vi "HTTP URL Format.vi"(3 "Endpoint":string="/Status", 4 "Port":string="11200", 5 "IP Address":string="10.0.40.4") -> (2 "URL":string)   [LabVIEW 2020]
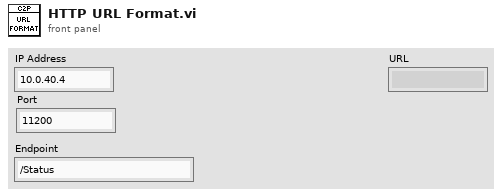
[diagram p1: front panel]
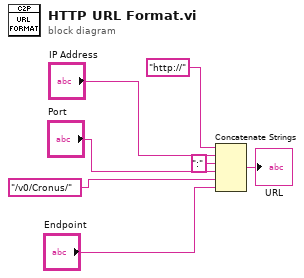
[diagram p0: block diagram]
diagram:
  n1 = Concatenate Strings("http://" ("url"), "IP Address", ":" ("string"), "Port", "/v0/Cronus/" ("url"), "Endpoint") -> (→"URL":string)
